vi "Tosca-Start Threads.vi"(0 "Uses vision":bool, 9 "IPC":T1, 11 "error in (no error)":errorcluster) -> (15 "error out":errorcluster)   [LabVIEW 2020]
uses:
  IPC VIs/Tosca-IPC.ctl
  Classes/Parameters/Parameters.lvclass
  Digital Input VIs/Tosca-DI Queue Data.ctl
  Digital Input VIs/Tosca-Input Event.ctl
  Digital Input VIs/Tosca-Input Criterion.ctl
  epl-vi-lib/Utility VIs/Type Defs/Logic State.ctl
  Typedefs/Tosca-Accumulator.ctl
  Typedefs/Tosca-State AODO.ctl
  Typedefs/Tosca-AO Runtime.ctl
  Typedefs/Tosca-DO Runtime.ctl
  epl-vi-lib/Signal Synthesis VIs/4th Generation/Classes/SignalManager/SignalManager.lvclass
  Typedefs/Tosca-Synapse Start Data.ctl
  IPC VIs/Tosca-Message.ctl
  IPC VIs/Tosca-Message Action.ctl
  Typedefs/Tosca-Thread Type.ctl
  Imaging VIs/Tosca-2P-Notifier Data.ctl
  Typedefs/Tosca-MATLAB Queue Data.ctl
  Visual Stim VIs/Tosca-Grating.ctl
  Visual Stim VIs/Tosca-Grating Type.ctl
  Typedefs/Tosca-File IO Notification.ctl
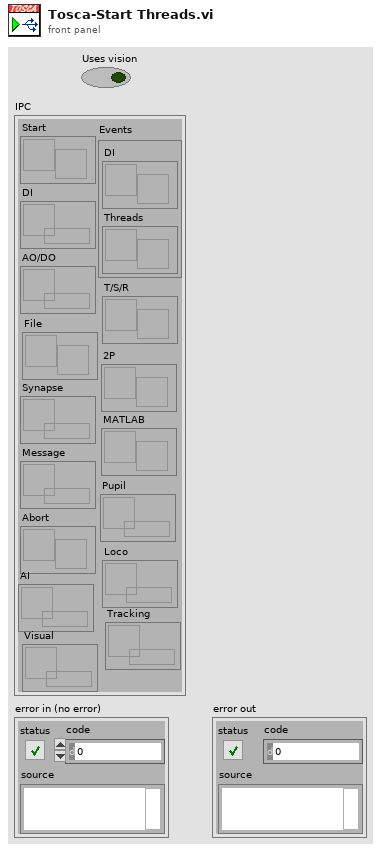
[diagram p1: front panel]
types:
  T1 = typedef "Tosca-IPC.ctl" = cluster{"Start":refnum<notifier>, "DI":refnum<queue>, "AO/DO":refnum<queue>, "Synapse":refnum<queue>, "Message":refnum<queue>, "Abort":refnum<notifier>, "Events":cluster{"DI":refnum<user-event>, "Threads ":refnum<user-event>}, "T/S/R":refnum<notifier>, "2P":refnum<notifier>, "MATLAB":refnum<notifier>, "Pupil":refnum<queue>, "Loco":refnum<queue>, "AI":refnum<queue>, "Tracking":refnum<queue>, "Visual":refnum<queue>, "File":refnum<notifier>}
  T2 = typedef "Tosca-Grating.ctl" = cluster{"Type":T3, "Orientation (deg)":dbl, "Spatial frequency (cpd)":dbl, "Velocity (Hz)":dbl, "Contrast":dbl, "Background intensity":dbl, "Duration (ms)":dbl, "Phase (cycles)":dbl}
  T3 = typedef "Tosca-Grating Type.ctl" = enum16{"OFF", "Square", "Sine"}
  T4 = typedef "Tosca-Visual Display Settings.ctl" = cluster{"Use PTB":bool, "IP Address":string, "Port":i32, "rect":cluster{"left":i16, "top":i16, "width":i16, "height":i16}, "Full screen":bool, "Open at start":bool, "Monitor":i32, "Monitor size (in)":dbl, "Monitor dist (in)":dbl, "Photodiode Square":cluster{"size":i16, "location":enum16{"Bottom Left", "Top Left", "Top Right", "Bottom Right"}}, "Background":dbl}
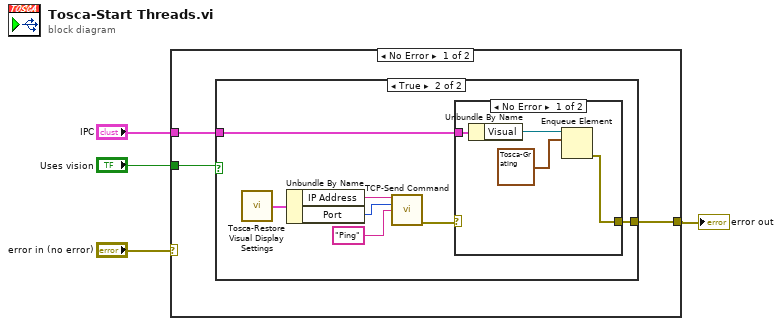
[diagram p0: block diagram]
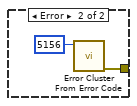
[diagram p3: hidden frame]
diagram:
  n1 = case shown="No Error" "error in (no error)" {
    selector: "error in (no error)" -> [_ w21]
    tunnel: "IPC" -> [w7 _]
    tunnel: [w6 w21] -> w2
    tunnel: "Uses vision" -> [w5 _]
    frame No Error {
      n2 = case shown="True" w5 {
        tunnel: w7 -> [_ w14]
        tunnel: [_ w12] -> w6
        frame False {
        }
        frame True {
          n3 = call "Tosca-Restore Visual Display Settings.vi"() -> ("Visual Display Settings"=w13:T4)  [unwired: 14 in, 1 out]
          n4 = Unbundle By Name(w13) -> ("IP Address"=w11:string, "Port"=w10:i32)
          n5 = call "TCP-Send Command.vi"("PXI Address"=w11, "Port"=w10, "Command"="Ping") -> ("error out"=w9:errorcluster)  [unwired: 12 in]
          n6 = case shown="No Error" w9 {
            tunnel: w14 -> [w18 _]
            tunnel: [w15 w20] -> w12
            frame No Error {
              n7 = Unbundle By Name(w18) -> ("Visual"=w17:refnum<queue>)
              n8 = Enqueue Element(queue=w17, element=T2 {"Type"=enum."OFF", "Orientation (deg)"=0.0, "Spatial frequency (cpd)"=0.0, "Velocity (Hz)"=0.0, "Contrast"=0.0, "Background intensity"=0.0, "Duration (ms)"=0.0, "Phase (cycles)"=0.0}) -> (error out=w15:errorcluster)  [unwired: 2 in, 2 out]
            }
            frame Error {
              n9 = call <vilib>:"Error Cluster From Error Code.vi"("error code (0)"=5156) -> ("error out"=w20:errorcluster)  [unwired: 8 in]
            }
          }
        }
      }
    }
    frame Error {
    }
  }
  "error out" <- w2
